vi "GetType.vi"(8 "error in (no error)":errorcluster, 11 "Set Output Lines Msg":refnum<class "Set Output Lines Msg.lvclass">) -> (0 "error out":errorcluster, 2 "Data Sample":variant, 3 "Set Output Lines Msg":refnum<class "Set Output Lines Msg.lvclass">)   [LabVIEW 2020, in "BNT_ULx.lvlib" / "Set Output Lines Msg.lvclass"]
uses:
  Set Output Lines Msg.lvclass
  Set Output Lines Msg.lvclass/Set Output Lines Msg.ctl
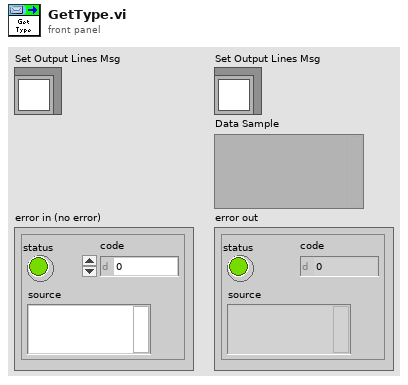
[diagram p1: front panel]
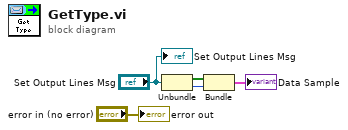
[diagram p0: block diagram]
diagram:
  n1 = Unbundle("Set Output Lines Msg") -> (w2:bool[], w1:i32)
  n2 = Bundle("DO Lines"=w2, "Start Index"=w1) -> (→"Data Sample":cluster{"DO Lines":bool[], "Start Index":i32})  [unwired: 1 in]
  "error out" <- "error in (no error)"
  "Set Output Lines Msg" <- "Set Output Lines Msg"
